vi "getSignalOut.vi"(6 "Delay between send and receive [ms]":i32=100, 8 "error in (no error)":errorcluster, 11 "CCD in":refnum<class "CCD.lvclass">) -> (0 "error out":errorcluster, 3 "CCD out":refnum<class "CCD.lvclass">)   [LabVIEW 2023, in "CCD.lvclass"]
uses:
  CCD.lvclass
  CCD.lvclass/CCD.ctl
  20f7d3bd-08ac-4524-9bed-df36c1da25a0.vi
  a21955fc-e3a0-4e36-8495-41f1bfac7860.vi
  GenericDevice/GenericDevice.lvclass
panel:
  # "Connector Pane"
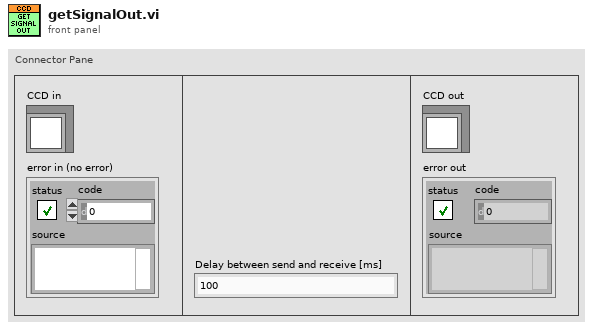
[diagram p1: front panel]
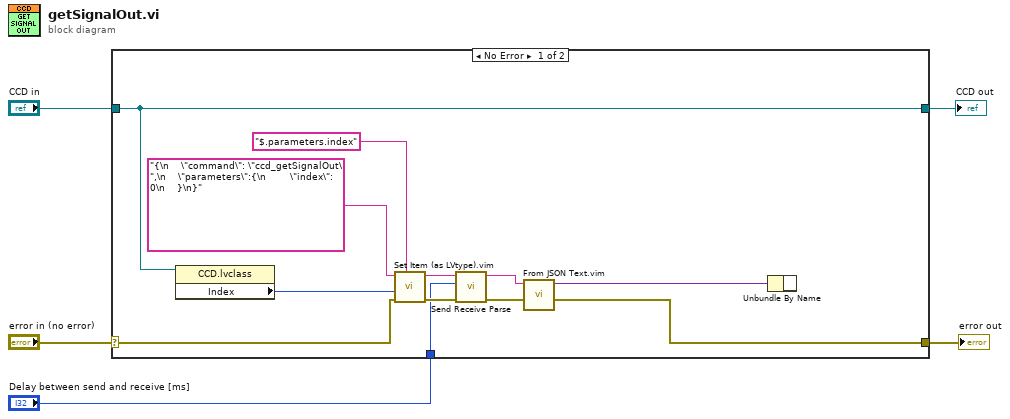
[diagram p0: block diagram]
diagram:
  n1 = case shown="No Error" "error in (no error)" {
    selector: "error in (no error)" -> [w13 w19]
    tunnel: [w12 w19] -> w4
    tunnel: [w15 w18] -> w2
    tunnel: "CCD in" -> [w15 w18]
    tunnel: "Delay between send and receive [ms]" -> [w6 _]
    frame No Error {
      n2 = property class="CCD.lvclass"(reference=w15) -> ("Index"=w14:i32)  [unwired: 1 in, 2 out]
      n3 = call "Set Item (as LVtype).vim"("$Path or Item Name"="$.parameters.index", "error in (no error)"=w13, "Anything"=w14, "JSON"="{\n    \"command\": \"ccd_getSignalOut\",\n    \"parameters\":{\n        \"index\": 0\n    }\n}") -> ("error out"=w9:errorcluster, "<JSON>"=w11:string)  [unwired: 4 in, 1 out]
      n4 = call "Send Receive Parse.vi"("error in"=w9, "Delay between send and receive [ms]"=w6, "<JSON>"=w11) -> ("error out"=w8:errorcluster, "results-JSON string"=w10:string)  [unwired: 6 in, 1 out]
      n5 = call "From JSON Text.vim"("error in (no error)"=w8, "JSON"=w10) -> ("error out"=w12:errorcluster, "Data out"=w7:variant)  [unwired: 8 in]
      n6 = Unbundle By Name(w7) -> ()  [unwired: 1 out]
    }
    frame Error {
    }
  }
  "error out" <- w4
  "CCD out" <- w2
